vi "WriteTreeStrict.vi"(8 "error in (no error)":errorcluster, 10 "Tree":refnum<vi>, 11 "ClassDataTree in":refnum<class "ClassDataTree.lvclass">) -> (0 "error out":errorcluster, 3 "ClassDataTree out":refnum<class "ClassDataTree.lvclass">)   [LabVIEW 2010, in "ClassDataTree.lvclass"]
uses:
  ClassDataTree.lvclass
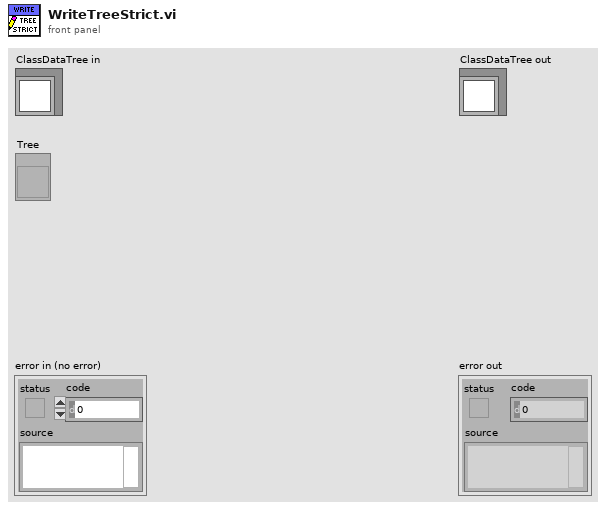
[diagram p1: front panel]
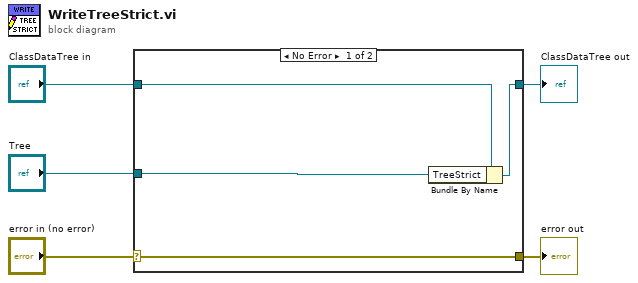
[diagram p0: block diagram]
diagram:
  n1 = case shown="No Error" "error in (no error)" {
    selector: "error in (no error)" -> [w9 w10]
    tunnel: [w9 w10] -> w4
    tunnel: [w7 w11] -> w2
    tunnel: "ClassDataTree in" -> [w8 w11]
    tunnel: "Tree" -> [w6 _]
    frame No Error {
      n2 = Bundle By Name(cluster=w8, "TreeStrict"=w6) -> (w7:refnum<class "ClassDataTree.lvclass">)
    }
    frame Error {
    }
  }
  "error out" <- w4
  "ClassDataTree out" <- w2
